vi "decodeStream.vi"(8 "error in (no error)":errorcluster, 9 "beginIndex":i32, 10 "binary stream":u8[](array[numeric]), 11 "tBSONDouble in":refnum<class "tBSONDouble.lvclass">) -> (0 "error out":errorcluster, 1 "endIndex":i32, 2 "binary stream out":u8[](array[numeric]), 3 "tBSONDouble out":refnum<class "tBSONDouble.lvclass">)   [LabVIEW 2013, in "BSON.lvlib" / "tBSONDouble.lvclass"]
uses:
  tBSONDouble.lvclass
  tBSONElement/tBSONElement.lvclass
  status.ctl
  setValue.vi
  BSON.lvlib
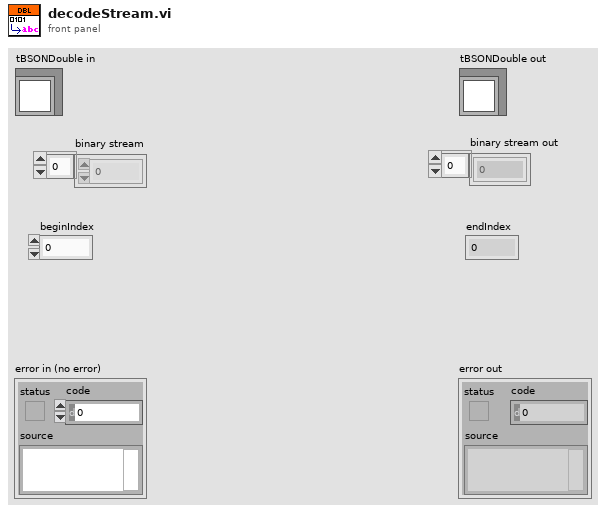
[diagram p1: front panel]
types:
  T1 = typedef "BSON.lvlib/status.ctl" = enum16{"Stream Corrupted or Ended Abruptly", "Incorrect Type In Stream", "ObjectID Invalid", "Method Not Implemented", "Invalid Name", "Invalid URI", "AutoReconnect", "Operation Failed", "Incorrectly Configured", "Cursor Not Found", "Timeout", "Invalid Type", "Empty Name", "Duplicate Name", "MD5Incorrect"}
  T2 = enum16{"big-endian, network order", "native, host order", "little-endian"}
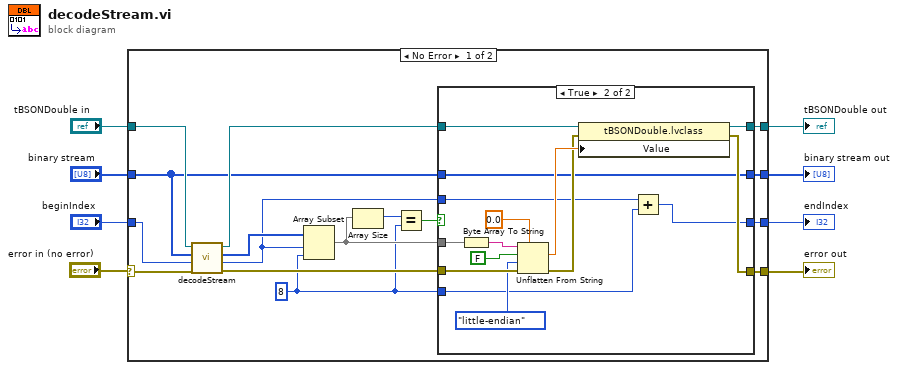
[diagram p0: block diagram]
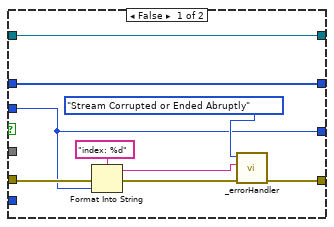
[diagram p2: hidden frame]
diagram:
  n1 = case shown="No Error" "error in (no error)" {
    selector: "error in (no error)" -> [w24 w52]
    tunnel: [w20 w52] -> w4
    tunnel: "beginIndex" -> [w22 w51]
    tunnel: [w12 w51] -> w3
    tunnel: "binary stream" -> [w11 w50]
    tunnel: [w10 w50] -> w2
    tunnel: "tBSONDouble in" -> [w23 w49]
    tunnel: [w19 w49] -> w1
    frame No Error {
      w9 = 8
      n2 = call-parent "decodeStream.vi"("error in (no error)"=w24, "beginIndex"=w22, "binary stream"=w11, "tBSONElement in"=w23) -> ("error out"=w15:errorcluster, "endIndex"=w13:i32, "binary stream out"=w18:u8[], "tBSONElement out"=w21:refnum<class "tBSONDouble.lvclass">)  [unwired: 4 in]
      n3 = Array Subset(array=w18, index=w13, length=w9) -> (w14:u8[])
      n4 = Array Size(array=w14) -> (size(s)=w17:i32)
      n5 = Equal?(x=w17, y=w9) -> (x = y?=w16:bool)
      n6 = case shown="True" w16 {
        tunnel: w21 -> [w25 w39]
        tunnel: [w28 w48] -> w20
        tunnel: [w25 w47] -> w19
        tunnel: w15 -> [w29 w44]
        tunnel: w14 -> [_ w46]
        tunnel: w13 -> [w27 w36]
        tunnel: [w27 w34] -> w12
        tunnel: w11 -> [w26 w37]
        tunnel: [w26 w37] -> w10
        tunnel: w9 -> [_ w35]
        frame False {
          n7 = Format Into String(format string="index: %d", error in=w29, w27) -> (resulting string=w32:string, error out=w31:errorcluster)  [unwired: 1 in]
          n8 = call "_errorHandler.vi"("error in (no error)"=w31, "Additional Text"=w32, "Error Type"=status."Stream Corrupted or Ended Abruptly") -> ("error out"=w28:errorcluster)  [unwired: 8 in]
        }
        frame True {
          n9 = Byte Array To String(unsigned byte array=w46) -> (string=w45:string)
          n10 = Unflatten From String(type=0.0, binary string=w45, data includes array or string size? (T)=FALSE, byte order (0:big-endian, network order)=T2."little-endian", error in (no error)=w44) -> (value=w40:dbl, error out=w38:errorcluster)  [unwired: 1 out]
          n11 = property class="tBSONDouble.lvclass"(reference=w39, error in=w38, "Value"=w40) -> (reference out=w47:refnum<class "tBSONDouble.lvclass">, error out=w48:errorcluster)
          n12 = Add(x=w36, y=w35) -> (x+y=w34:i32)
        }
      }
    }
    frame Error {
    }
  }
  "error out" <- w4
  "tBSONDouble out" <- w1
  "binary stream out" <- w2
  "endIndex" <- w3
